vi "Delete Last Element.vi"(8 "error in (no error)":errorcluster, 11 "Cluster in":variant) -> (0 "error out":errorcluster, 1 "element":variant, 2 "Name":string, 3 "Cluster out":variant)   [LabVIEW 2017, in "Variant Data Manipulation.lvlib"]
uses:
  Variant Data Manipulation.lvlib
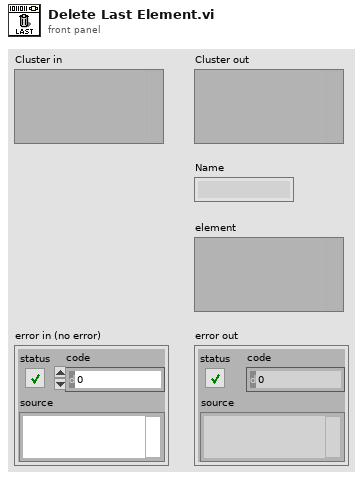
[diagram p1: front panel]
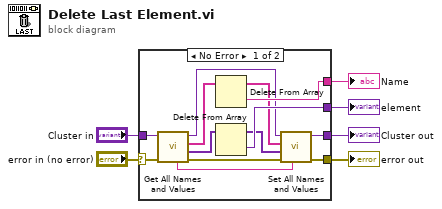
[diagram p0: block diagram]
diagram:
  n1 = case shown="No Error" "error in (no error)" {
    selector: "error in (no error)" -> [w19 w20]
    tunnel: [w16 w20] -> w5
    tunnel: [w15 w21] -> w4
    tunnel: "Cluster in" -> [w14 w21]
    tunnel: [w12 _] -> w2
    tunnel: [w11 _] -> w1
    frame No Error {
      n2 = call "Get All Names and Values.vi"("error in"=w19, "Cluster in"=w14) -> ("error out"=w17:errorcluster, "Values"=w18:variant[], "Element Names"=w13:string[], "Cluster out"=w7:variant, "Cluster Name"=w8:string)  [unwired: 5 in]
      n3 = Delete From Array(array=w13) -> (deleted portion=w12:string, array with subset deleted=w10:string[])  [unwired: 2 in]
      n4 = Delete From Array(array=w18) -> (deleted portion=w11:variant, array with subset deleted=w9:variant[])  [unwired: 2 in]
      n5 = call "Set All Names and Values.vi"("Cluster Name"=w8, "error in"=w17, "values"=w9, "Element Names"=w10, "Cluster in"=w7) -> ("error out"=w16:errorcluster, "Cluster out"=w15:variant)  [unwired: 5 in]
    }
    frame Error {
    }
  }
  "Cluster out" <- w4
  "error out" <- w5
  "element" <- w1
  "Name" <- w2
